vi "Speed Mode.vi"(8 "error in (no error)":errorcluster, 10 "String":string, 11 "High Speed in":refnum<class "High Speed.lvclass">) -> (0 "error out":errorcluster, 2 "This VI":refnum<vi>, 3 "High Speed out":refnum<class "High Speed.lvclass">)   [LabVIEW 2020, in "High Speed.lvclass"]
uses:
  High Speed.lvclass
  High Speed.lvclass/High Speed.ctl
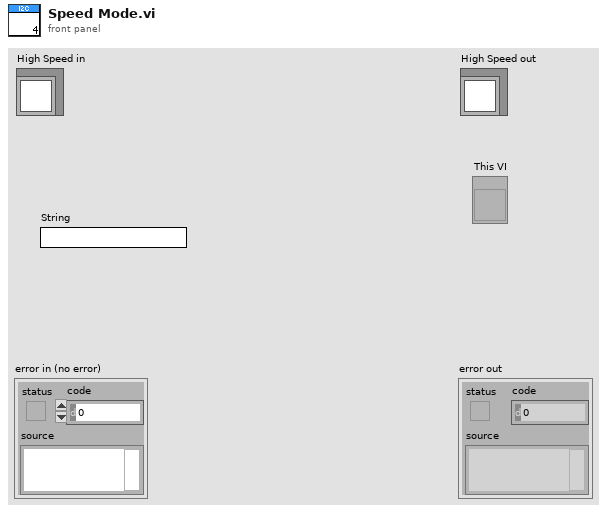
[diagram p1: front panel]
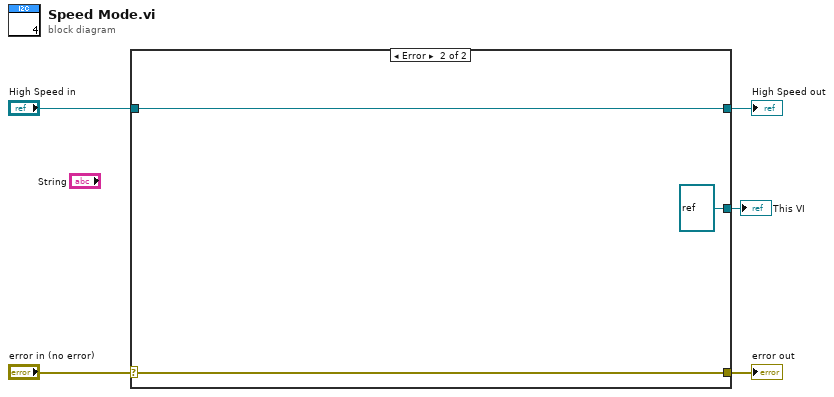
[diagram p0: block diagram]
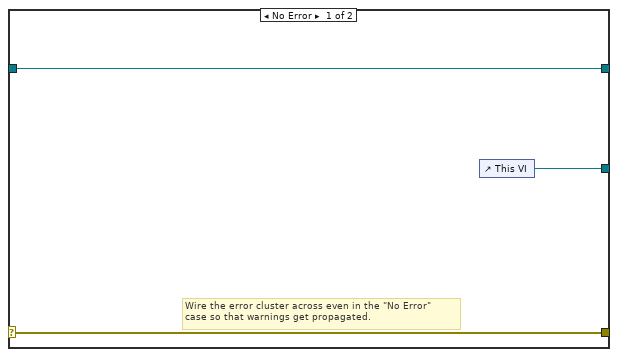
[diagram p2: hidden frame]
diagram:
  n1 = case shown="Error" "error in (no error)" {
    selector: "error in (no error)" -> [w7 w11]
    tunnel: [w7 w11] -> w4
    tunnel: [w8 w10] -> w2
    tunnel: "High Speed in" -> [w8 w10]
    tunnel: [w6 refnum<vi> refnum ("This VI")] -> w1
    frame No Error {
      # "Wire the error cluster across even in the \"No Error\"\ncase so that warnings get propagated."
      n2 = control-ref of="This VI"() -> (w6:refnum<vi>)
    }
    frame Error {
    }
  }
  "error out" <- w4
  "High Speed out" <- w2
  "This VI" <- w1
